vi "Result.Load Test Limits from JSON File.vi"(8 "error in (no error)":errorcluster, 9 "JSON to Data Names":string[][](array[string]), 11 "Limit File Path":path) -> (0 "error out":errorcluster, 1 "Limits":T1[](array[typedef])=[{"Name"="asv", "LimType"=enum."None", "LL"="", "UL"="", "Units"="", "FailCode"=0, "FailDesc"=""}, {"Name"=", kjh/lk", "LimType"=enum."None", "LL"="", "UL"="", "Units"="", "FailCode"=0, "FailDesc"=""}], 2 "File Version":string, 3 "File Name":string, 4 "Limits in Variant":variant, 5 "FaultCode Prefix":i32)   [LabVIEW 2019]
uses:
  <vilib>/KATE/Files/File Utils.lvlib
  Result.Limit Type.ctl
  Limits/Result.Test Limit Item.ctl
panel:
  out "Test Name":string
  out "XML Version":string
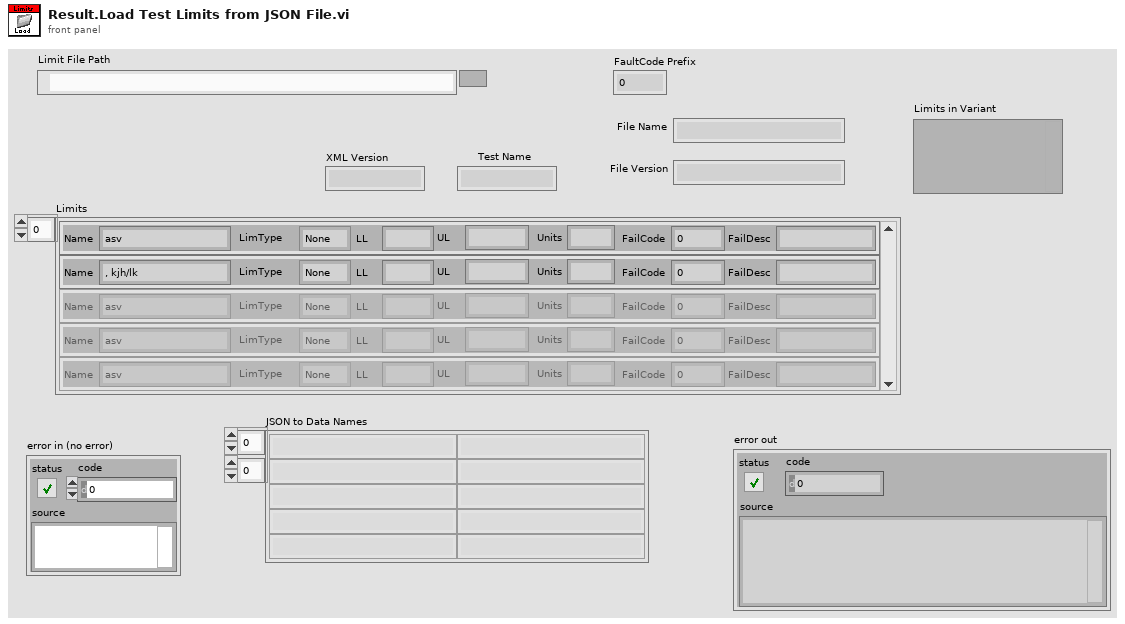
[diagram p1: front panel]
types:
  T1 = typedef "Result.Test Limit Item.ctl" = cluster{"Name":string, "LimType":T2, "LL":string, "UL":string, "Units":string, "FailCode":i32, "FailDesc":string}
  T2 = typedef "Result.Limit Type.ctl" = enum16{"None", "EQ", "NE", "GT", "LT", "GE", "LE", "GTLT", "GELE", "GELT", "GTLE", "LTGT", "LEGE", "LEGT", "LTGE", "Contains", "NotContains"}
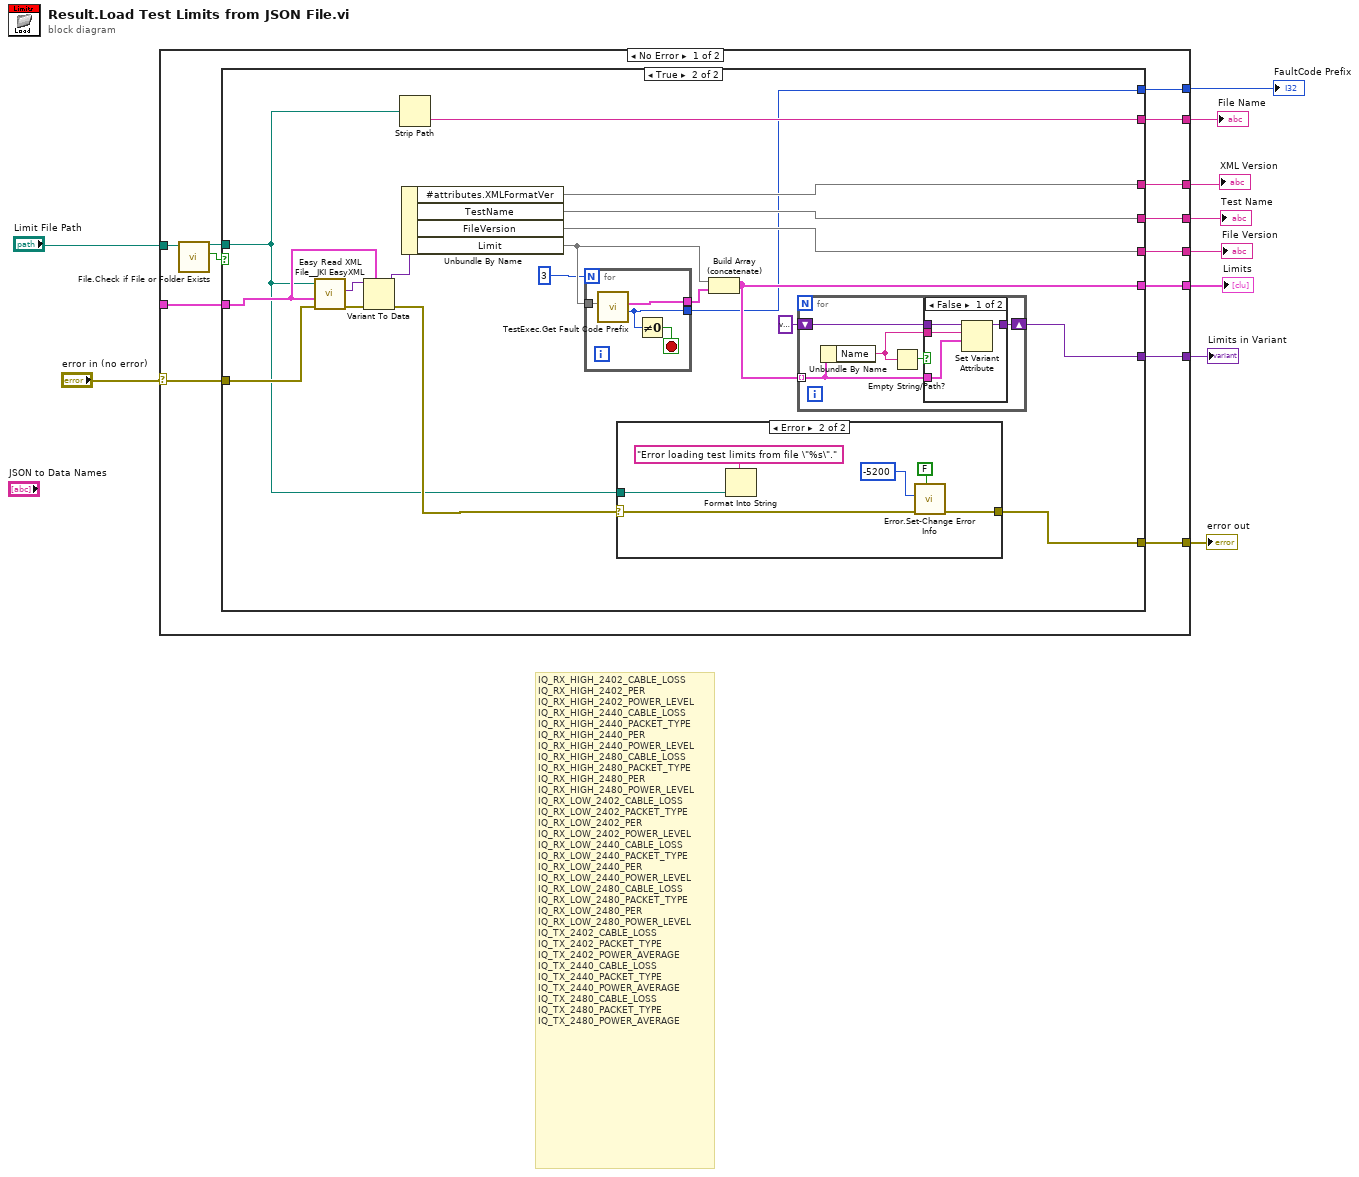
[diagram p0: block diagram]
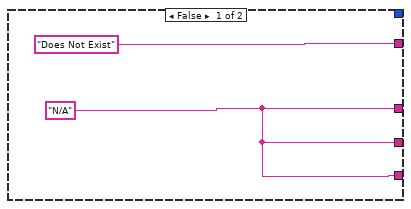
[diagram p2: hidden frame]
diagram:
  # "IQ_RX_HIGH_2402_CABLE_LOSS\nIQ_RX_HIGH_2402_PER\nIQ_RX_HIGH_2402_POWER_LEVEL\nIQ_RX_HIGH_2440_CABLE_LOSS\nIQ_RX_HIGH_2440_PACKET_TYPE\nIQ_RX_HIGH_2440_PER\nIQ_RX_HIGH_2440_POWER_LEVEL\nIQ_RX_HIGH_2480_CABLE_LOSS\nIQ_RX_HIGH_2480_PACKET_TYPE\nIQ_RX_HIGH_2480_PER\nIQ_RX_HIGH_2480_POWER_LEVEL\nIQ_RX_LOW_2402_CABLE_LOSS\nIQ_RX_LOW_2402_PACKET_TYPE\nIQ_RX_LOW_2402_PER\nIQ_RX_LOW_2402_POWER_LEVEL\nIQ_RX_LOW_2440_CABLE_LOSS\nIQ_RX_LOW_2440_PACKET_TYPE\nIQ_RX_LOW_2440_PER\nIQ_RX_LOW_2440_POWER_LEVEL\nIQ_RX_LOW_2480_CABLE_LOSS\nIQ_RX_LOW_2480_PACKET_TYPE\nIQ_RX_LOW_2480_PER\nIQ_RX_LOW_2480_POWER_LEVEL\nIQ_TX_2402_CABLE_LOSS\nIQ_TX_2402_PACKET_TYPE\nIQ_TX_2402_POWER_AVERAGE\nIQ_TX_2440_CABLE_LOSS\nIQ_TX_2440_PACKET_TYPE\nIQ_TX_2440_POWER_AVERAGE\nIQ_TX_2480_CABLE_LOSS\nIQ_TX_2480_PACKET_TYPE\nIQ_TX_2480_POWER_AVERAGE"
  n1 = case shown="No Error" "error in (no error)" {
    selector: "error in (no error)" -> [w17 w67]
    tunnel: [w24 _] -> w11
    tunnel: [w23 _] -> w10
    tunnel: [w22 _] -> w9
    tunnel: [w21 _] -> w8
    tunnel: [w20 _] -> w7
    tunnel: [w19 _] -> w6
    tunnel: [w18 _] -> w5
    tunnel: [w16 w67] -> w3
    tunnel: "Limit File Path" -> [w14 _]
    tunnel: [w12 _] -> w1
    frame No Error {
      n2 = call <vilib>:"File.Check if File or Folder Exists.vi"("Path"=w14) -> ("Exists"=w13:bool, "Dup Path"=w15:path)  [unwired: 6 in, 3 out]
      n3 = case shown="True" w13 {
        tunnel: w24 -> [_ w42]
        tunnel: [w25 w41] -> w23
        tunnel: [w25 w40] -> w22
        tunnel: [w25 w39] -> w21
        tunnel: ["Does Not Exist" w38] -> w20
        tunnel: [_ w31] -> w19
        tunnel: [_ w36] -> w18
        tunnel: w17 -> [_ w35]
        tunnel: [_ w33] -> w16
        tunnel: w15 -> [_ w32]
        tunnel: [_ w29] -> w12
        frame False {
          w25 = "N/A"
        }
        frame True {
          n4 = call <vilib>:"Easy Read XML File__JKI EasyXML.vi"("error in (no error)"=w35, "LabVIEW Data (Type)"=w42, "XML File Path"=w32) -> ("error out"=w45:errorcluster, "LabVIEW Data"=w44:variant)  [unwired: 6 in, 1 out]
          n5 = Variant To Data(error in=w45, type=w42, Variant=w44) -> (data=w43:variant, error out=w34:errorcluster)
          n6 = Strip Path(path=w32) -> (name=w38:string)  [unwired: 1 out]
          n7 = Unbundle By Name(w43) -> ("#attributes.XMLFormatVer"=w41, "TestName"=w40, "FileVersion"=w39, "Limit"=w30)
          n8 = for {
            N: 3 -> [_]
            tunnel: w30 -> [w49]
            tunnel: [w47] -> w29
            tunnel: [w48] -> w28
            stop <- w46 stop-if-true
            n9 = call "TestExec.Get Fault Code Prefix.vi"("Limit In"=w49) -> ("FaultCode Prefix"=w47:i32, "Code Prefix Lim Out"=w48:T1)  [unwired: 9 in]
            n10 = Not Equal To 0?(x=w47) -> (x != 0?=w46:bool)
          }
          n11 = case shown="Error" w34 {
            selector: w34 -> [w50 w56]
            tunnel: [w50 w54] -> w33
            tunnel: w32 -> [_ w52]
            frame No Error {
            }
            frame Error {
              n12 = Format Into String(format string="Error loading test limits from file \"%s\".", w52) -> ()  [unwired: 2 in, 2 out]
              n13 = call "Error.Set-Change Error Info.vi"("Append Details"=FALSE, "error in"=w56, "Cust Code(0 = no change)"=-5200 ("code")) -> ("error out"=w54:errorcluster)  [unwired: 8 in]
            }
          }
          n14 = Build Array (concatenate)(w30, w28) -> (w31:T1[])
          n15 = for {
            tunnel: w31 -> [w59] mode=indexing
            shift-right: [w60] -> w36
            shift-left: variant ("Limits in Variant") -> [w61]
            n16 = Unbundle By Name(w59) -> ("Name"=w58:string)
            n17 = Empty String/Path?(string/path=w58) -> (empty?=w57:bool)
            n18 = case shown="False" w57 {
              tunnel: w61 -> [w65 w66]
              tunnel: [w64 w66] -> w60
              tunnel: w59 -> [w63 _]
              tunnel: w58 -> [w62 _]
              frame False {
                n19 = Set Variant Attribute(Variant=w65, name=w62, value=w63) -> (Variant out=w64:variant)  [unwired: 1 in, 2 out]
              }
              frame True {
              }
            }
          }
        }
      }
    }
    frame Error {
    }
  }
  "Limits" <- w6
  "XML Version" <- w10
  "File Name" <- w7
  "File Version" <- w8
  "Test Name" <- w9
  "Limits in Variant" <- w5
  "error out" <- w3
  "FaultCode Prefix" <- w1
